vi "Update Subsystem.vi"(8 "error in (no error)":errorcluster, 9 "New Owner":refnum<class "Attribute.Owner.lvclass">, 10 "Current Identity":refnum<class "Attribute.Identity.lvclass">) -> (0 "error out":errorcluster, 2 "Updated Identity":refnum<class "Attribute.Identity.lvclass">)   [LabVIEW 2021, in "smo.lvlib" / "Registry-SMO.lvclass"]
uses:
  Registry-SMO.lvclass
  Support/Attribute.Owner/Attribute.Owner.lvclass
  Support/Attribute.Identity/Attribute.Identity.lvclass
  SMO_Info--Cluster.ctl
  Support/Attribute.Owner/Attribute.Owner.lvclass/Attribute.Owner.ctl
  Support/Attribute.Identity/Attribute.Identity.lvclass/Attribute.Identity.ctl
  Registry-SMO.lvclass/Registry-SMO.ctl
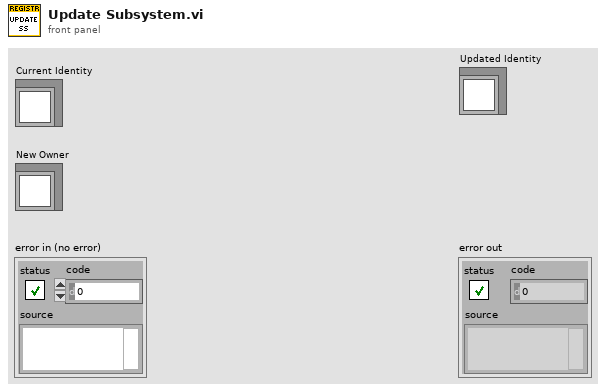
[diagram p1: front panel]
types:
  T1 = typedef "smo.lvlib/Registry-SMO.lvclass/SMO_Info--Cluster.ctl" = cluster{"Name":string, "Shared Resource":bool}
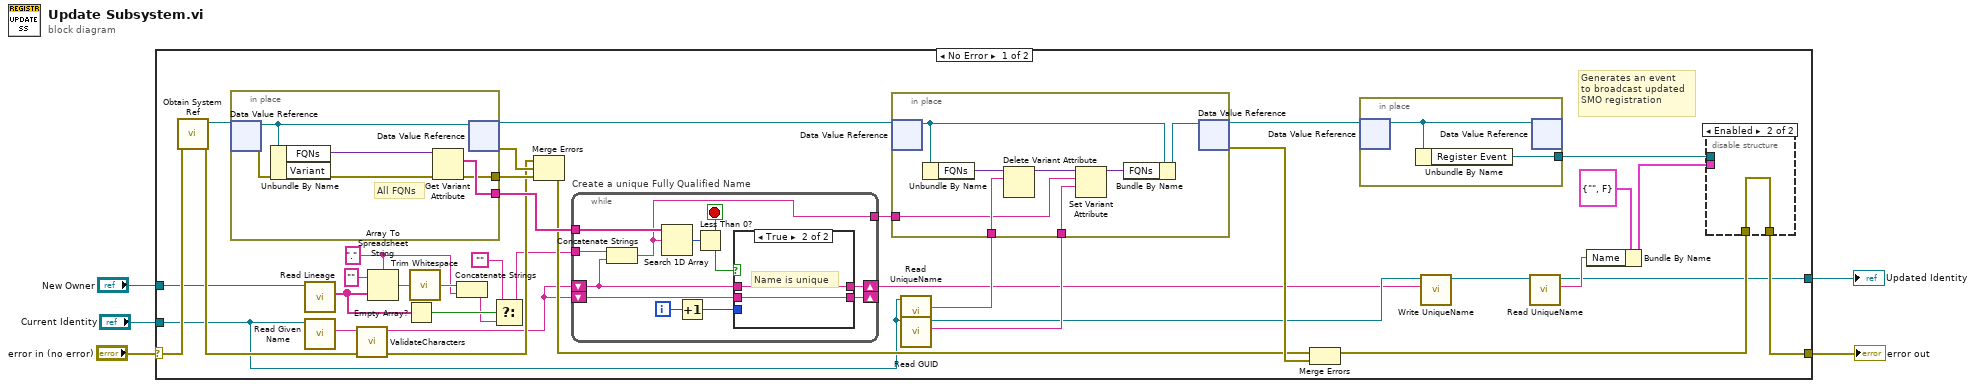
[diagram p0: block diagram]
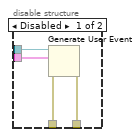
[diagram p2: hidden frame]
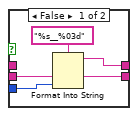
[diagram p3: hidden frame]
diagram:
  n1 = case shown="No Error" "error in (no error)" {
    selector: "error in (no error)" -> [w40 w80]
    tunnel: [w29 w80] -> w4
    tunnel: "New Owner" -> [w19 _]
    tunnel: [w23 w79] -> w2
    tunnel: "Current Identity" -> [w20 w79]
    frame No Error {
      w14 = "." ("delimiter (Tab)")
      # "Generates an event\nto broadcast updated\nSMO registration"
      n2 = call "Obtain System Ref.vi"("error in (no error)"=w40) -> ("error out"=w34:errorcluster, "JKI SMO System"=w39:refnum<data-value>)  [unwired: 9 in]
      n3 = in-place {
        in-place-border: [w68] -> w38
        in-place-border: [w67] -> w35
        # "All FQNs"
        n4 = in-place-dvr #1(w39) -> (w66:refnum<class "Registry-SMO.lvclass">, w69:errorcluster)
        n5 = Unbundle By Name(w66) -> ("FQNs"=w70:variant)  [unwired: 1 out]
        n6 = Get Variant Attribute(Variant=w70, error in=w69) -> (names=w68:string[], error out=w67:errorcluster)  [unwired: 2 in, 2 out]
        n7 = in-place-dvr #1(w66) -> (w37:refnum<data-value>, w36:errorcluster)
      }
      n8 = call "Read Lineage.vi"("Attribute.Owner in"=w19) -> ("Lineage"=w12:string[])  [unwired: 8 in, 2 out]
      n9 = call "Read Given Name.vi"("Attribute.Identity in"=w20) -> ("Given Name"=w17:string)  [unwired: 9 in, 1 out]
      n10 = call "ValidateCharacters.vi"("Subsystem Name (optional)"=w17) -> ("Validated characters"=w13:string)  [unwired: 10 in]
      n11 = Array To Spreadsheet String(delimiter (Tab)=w14, array=w12, 3:"" ("format string")) -> (spreadsheet string=w16:string)
      n12 = Empty Array?(array=w12) -> (empty?=w11:bool)
      n13 = call <vilib>:"Trim Whitespace.vi"("string"=w16) -> ("trimmed string"=w15:string)  [unwired: 1 in]
      n14 = Concatenate Strings(w15, w14) -> (w10:string)
      n15 = Select(t="", s=w11, f=w10) -> (s? t:f=w9:string)
      n16 = Merge Errors(w34, w36, w35) -> (w33:errorcluster)
      n17 = while "Create a unique Fully Qualified Name" {
        tunnel: w38 -> [w59]
        shift-right: [w56] -> w7
        shift-left: w13 -> [w50]
        shift-right: [w52] -> _
        shift-left: w13 -> [w55]
        tunnel: w9 -> [w51]
        tunnel: [w49] -> w6
        i -> [w54]
        stop <- w57 stop-if-true
        n18 = Concatenate Strings(w51, w50) -> (w49:string)
        n19 = Search 1D Array(1D array=w59, element=w49) -> (index of element=w58:i32)  [unwired: 1 in]
        n20 = Increment(x=w54) -> (x+1=w53:i32)
        n21 = Less Than 0?(x=w58) -> (x < 0?=w57:bool)
        n22 = case shown="True" w57 {
          tunnel: w50 -> [_ w65]
          tunnel: [w63 w65] -> w56
          tunnel: w55 -> [w60 w64]
          tunnel: w53 -> [w62 _]
          tunnel: [w60 w64] -> w52
          frame False {
            n23 = Format Into String(format string="%s__%03d", w60, w62) -> (resulting string=w63:string)  [unwired: 2 in, 1 out]
          }
          frame True {
            # "Name is unique"
          }
        }
      }
      n24 = call "Read UniqueName.vi"("Attribute.Identity in"=w20) -> ("Unique Name"=w26:string)  [unwired: 9 in, 1 out]
      n25 = call "Read GUID.vi"("Attribute.Identity in"=w20) -> ("GUID"=w27:string, "Attribute.Identity out"=w22:refnum<class "Attribute.Identity.lvclass">)  [unwired: 8 in, 1 out]
      n26 = in-place {
        in-place-border: w27 -> [w75]
        in-place-border: w26 -> [w72]
        in-place-border: w6 -> [w71]
        n27 = in-place-dvr #2(w37) -> (w77:refnum<class "Registry-SMO.lvclass">)  [unwired: 1 out]
        n28 = Unbundle By Name(w77) -> ("FQNs"=w74:variant)
        n29 = Delete Variant Attribute(6:w72, 7:w74) -> (3:w73:variant)  [unwired: 1 in, 2 out]
        n30 = Set Variant Attribute(Variant=w73, name=w71, value=w75) -> (Variant out=w76:variant)  [unwired: 1 in, 2 out]
        n31 = Bundle By Name(cluster=w77, "FQNs"=w76) -> (w78:refnum<class "Registry-SMO.lvclass">)
        n32 = in-place-dvr #2(w78) -> (w25:refnum<data-value>, w41:errorcluster)
      }
      n33 = Merge Errors(w33, w41) -> (w24:errorcluster)
      n34 = in-place {
        in-place-border: [w47] -> w32
        n35 = in-place-dvr #3(w25) -> (w48:refnum<class "Registry-SMO.lvclass">)  [unwired: 1 out]
        n36 = Unbundle By Name(w48) -> ("Register Event"=w47:refnum<user-event>)
        n37 = in-place-dvr #3(w48) -> ()  [unwired: 2 out]
      }
      n38 = call "Write UniqueName.vi"("Unique Name"=w7, "Attribute.Identity in"=w22) -> ("Attribute.Identity out"=w21:refnum<class "Attribute.Identity.lvclass">)  [unwired: 9 in]
      n39 = call "Read UniqueName.vi"("Attribute.Identity in"=w21) -> ("Unique Name"=w28:string, "Attribute.Identity out"=w23:refnum<class "Attribute.Identity.lvclass">)  [unwired: 9 in]
      n40 = Bundle By Name(cluster=T1 {"Name"="", "Shared Resource"=FALSE} ("Cluster"), "Name"=w28) -> (w30:T1)
      n41 = disable-structure shown="Enabled" {
        disable-tunnel: w32 -> [w45 _]
        disable-tunnel: w30 -> [w44 _]
        disable-tunnel: [w43 w46] -> w29
        disable-tunnel: w24 -> [w42 w46]
        frame Disabled {
          n42 = Generate User Event(user event=w45, event data cluster=w44, error in=w42) -> (error out=w43:errorcluster)  [unwired: 1 in, 1 out]
        }
        frame Enabled {
        }
      }
    }
    frame Error {
    }
  }
  "error out" <- w4
  "Updated Identity" <- w2
